vi "Create Octree node boxes.vi"(2 "Colour (emission)":T1={"Red"=0.0, "Green"=1.0, "Blue"=0.0, "Alpha"=1.0}, 3 "Draw populated leaf nodes only":bool=TRUE, 4 "Octree nodes array":T2[](array[typedef])) -> (0 "Error out":errorcluster, 1 "Octree node boxes array":refnum<vi>[](array[refnum]))   [LabVIEW 2014]
uses:
  Typedefs/TreeNodeBox.ctl
  Typedefs/Quad.ctl
  <vilib>/Utility/miscctls.llb/LVRGBAColorTypeDef.ctl
  <vilib>/picture/3D Picture Control/Object/Create Object (drawable).vi
  <vilib>/picture/3D Picture Control/NI_3D Picture Control.lvlib
panel:
  # "PN 19/01/2015"
  # "Vertices"
  # "Edges"
  # "Unit normal"
  # "Edge unit normals"
  # "Vertices"
  # "Edges"
  # "Unit normal"
  # "Edge unit normals"
  # "Vertices"
  # "Edges"
  # "Unit normal"
  # "Edge unit normals"
  # "Vertices"
  # "Edges"
  # "Unit normal"
  # "Edge unit normals"
  # "Vertices"
  # "Edges"
  # "Unit normal"
  # "Edge unit normals"
  # "Vertices"
  # "Edges"
  # "Unit normal"
  # "Edge unit normals"
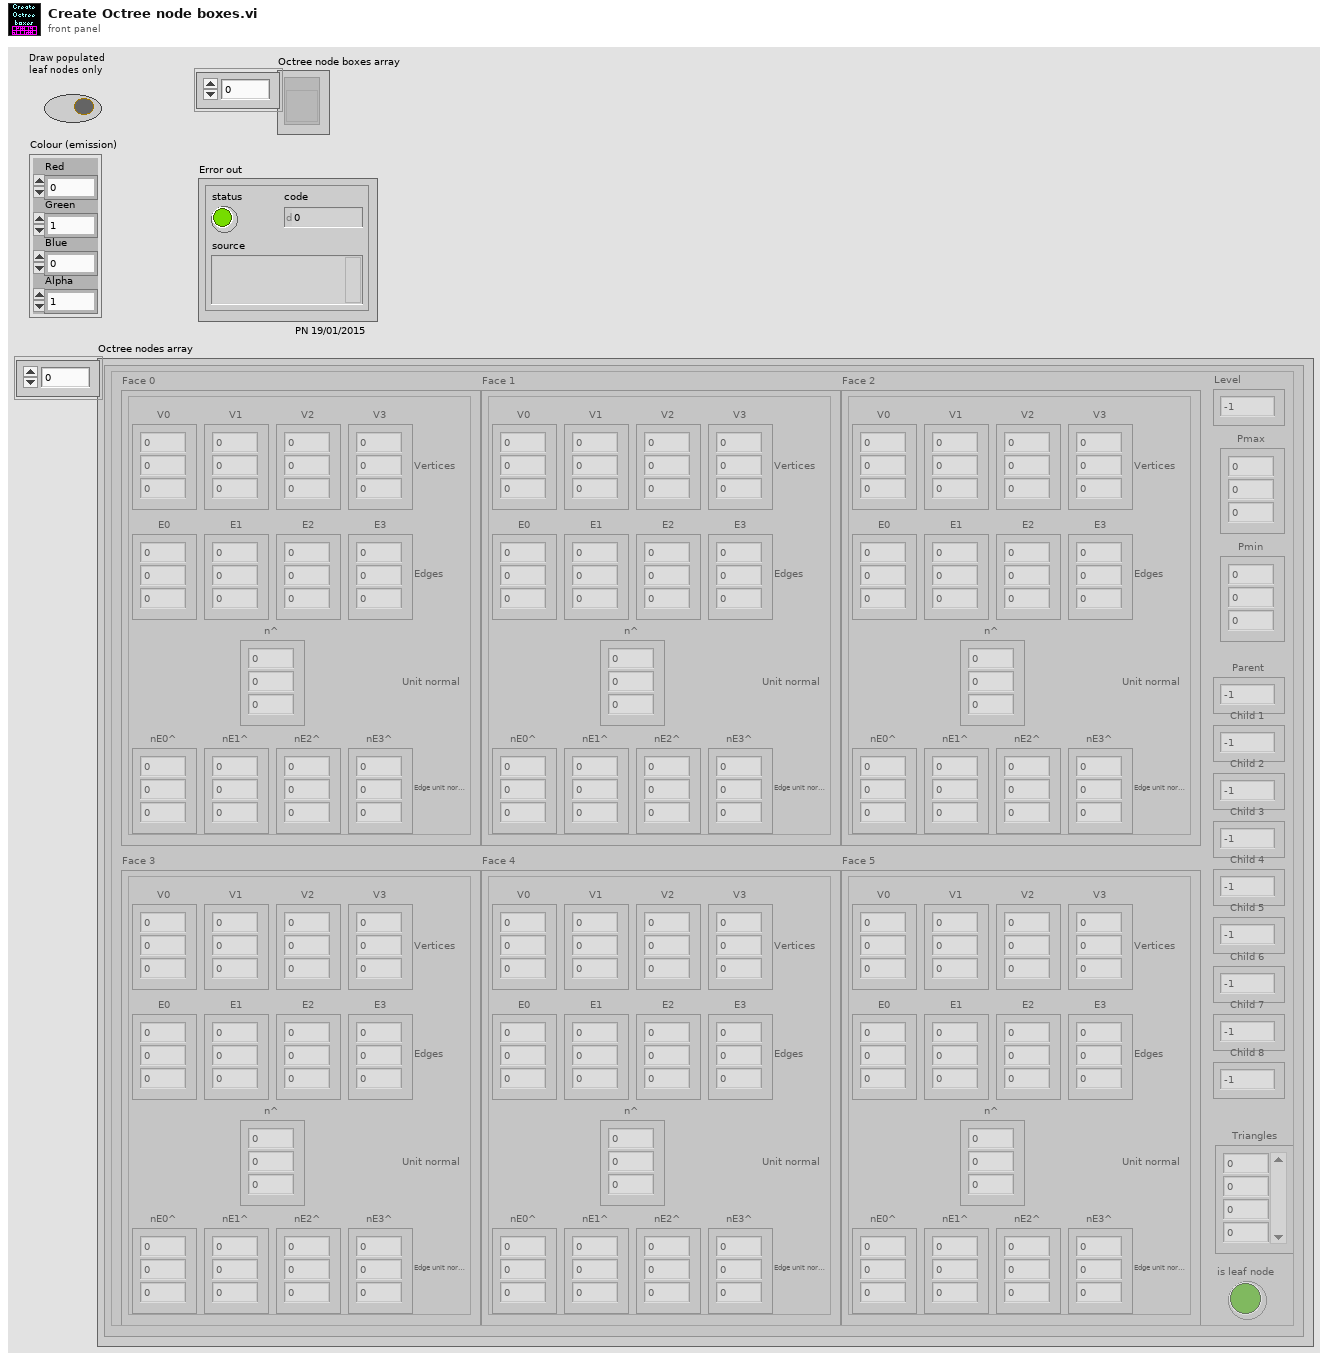
[diagram p1: front panel]
types:
  T1 = typedef "LVRGBAColorTypeDef.ctl" = cluster{"Red":sgl, "Green":sgl, "Blue":sgl, "Alpha":sgl}
  T2 = typedef "TreeNodeBox.ctl" = cluster{"Face 0":T3, "Face 1":T3, "Face 2":T3, "Face 3":T3, "Face 4":T3, "Face 5":T3, "Level":i32, "Pmax":sgl[], "Pmin":sgl[], "Parent":i32, "Child 1":i32, "Child 2":i32, "Child 3":i32, "Child 4":i32, "Child 5":i32, "Child 6":i32, "Child 7":i32, "Child 8":i32, "Triangles":i32[], "is leaf node":bool}
  T3 = typedef "Quad.ctl" = cluster{"V0":sgl[], "V1":sgl[], "V2":sgl[], "V3":sgl[], "E0":sgl[], "E1":sgl[], "E2":sgl[], "E3":sgl[], "n^":sgl[], "nE0^":sgl[], "nE1^":sgl[], "nE2^":sgl[], "nE3^":sgl[]}
  T4 = enum16{"Inherit Value", "Points", "Wireframe", "Polygons"}
  T5 = enum16{"Inherit Material", "Use entire Material", "Ignore Ambient", "Ignore Diffuse", "Ignore Specular", "Ignore Emission", "Ignore Ambient and Diffuse"}
  T6 = enum16{"Inherit Value", "No Culling", "Cull Back Face", "Cull Front Face", "Cull Both Faces"}
  T7 = enum16{"Inherit Value", "Counterclockwise", "Clockwise"}
  T8 = cluster{"Numeric":sgl, "Numeric":sgl, "Numeric":sgl}
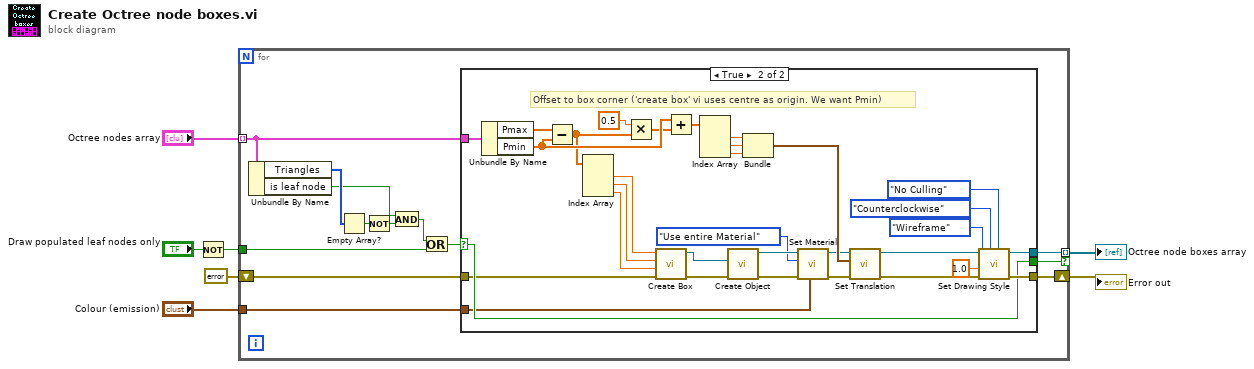
[diagram p0: block diagram]
diagram:
  n1 = Not(x="Draw populated leaf nodes only") -> (.not. x?=w6:bool)
  n2 = for {
    tunnel: "Octree nodes array" -> [w20] mode=indexing
    tunnel: w6 -> [w14]
    tunnel: [w12] -> w3 mode=indexing if=w10
    shift-right: [w11] -> w1
    shift-left: errorcluster {"status"=FALSE, "code"=0, "source"=""} ("error out") -> [w9]
    tunnel: "Colour (emission)" -> [w8]
    n3 = Unbundle By Name(w20) -> ("Triangles"=w19:i32[], "is leaf node"=w17:bool)
    n4 = Empty Array?(array=w19) -> (empty?=w18:bool)
    n5 = Not(x=w18) -> (.not. x?=w16:bool)
    n6 = And(x=w17, y=w16) -> (x .and. y?=w15:bool)
    n7 = Or(x=w15, y=w14) -> (x .or. y?=w13:bool)
    n8 = case shown="True" w13 {
      selector: w13 -> [w22 w32]
      tunnel: w20 -> [_ w54]
      tunnel: [_ w34] -> w12
      tunnel: [w21 w33] -> w11
      tunnel: [w22 w32] -> w10
      tunnel: w9 -> [w21 w31]
      tunnel: w8 -> [_ w25]
      frame False {
      }
      frame True {
        # "Offset to box corner ('create box' vi uses centre as origin. We want Pmin)"
        n9 = Unbundle By Name(w54) -> ("Pmax"=w44:sgl[], "Pmin"=w39:sgl[])
        n10 = Subtract(x=w44, y=w39) -> (x-y=w38:sgl[])
        n11 = Index Array(array=w38) -> (element #1=w43:sgl, element #2=w42:sgl, element #3=w41:sgl)  [unwired: 3 in]
        n12 = Multiply(x=sgl 0.5 ("Numeric"), y=w38) -> (x*y=w36:sgl[])
        n13 = call <vilib>:"Create Box.vi"("error in (no error)"=w31, "Length Z"=w41, "Length Y"=w42, "Length X"=w43) -> ("error out"=w52:errorcluster, "New Box Refnum"=w53:refnum<vi>)  [unwired: 6 in]
        n14 = Add(x=w39, y=w36) -> (x+y=w35:sgl[])
        n15 = Index Array(array=w35) -> (element #1=w47:sgl, element #2=w46:sgl, element #3=w45:sgl)  [unwired: 3 in]
        n16 = call-poly <vilib>:"Create Object.vi"("error in (no error)"=w52, "Geometry"=w53) -> ("error out"=w26:errorcluster, "Scene:New Object"=w30:refnum<vi>)  [unwired: 8 in]
        n17 = Bundle("Numeric"=w47, "Numeric"=w46, "Numeric"=w45) -> (w40:T8)  [unwired: 1 in]
        n18 = call <vilib>:"Set Material.vi"("Emission"=w25, "error in (no error)"=w26, "Color Mode"=T5."Use entire Material", "Scene Object In"=w30) -> ("error out"=w28:errorcluster, "Scene Object Out"=w29:refnum<vi>)  [unwired: 6 in]
        n19 = call <vilib>:"Set Translation.vi"("error in (no error)"=w28, "Translation"=w40, "Scene Object"=w29) -> ("error out"=w48:errorcluster, "Translated Object"=w49:refnum<vi>)  [unwired: 7 in]
        n20 = call <vilib>:"Set Drawing Style.vi"("Face Culling Mode"=T6."No Culling", "Frontface Mode"=T7."Counterclockwise", "error in (no error)"=w48, "Size"=1.0, "Mode"=T4."Wireframe", "Scene Object In"=w49) -> ("error out"=w33:errorcluster, "Scene Object Out"=w34:refnum<vi>)  [unwired: 4 in]
      }
    }
  }
  "Octree node boxes array" <- w3
  "Error out" <- w1
